vi "SubPanel_RunVI_Parameter.vi"(8 "error in (no error)":errorcluster, 9 "Values":variant[](array[variant]), 10 "Control Names":string[](array[string]), 11 "VIref in":refnum<vi>) -> (0 "error out":errorcluster, 3 "VIref out":refnum<vi>)   [LabVIEW 2014, in "SubPanelModule.lvlib"]
doc: "Imposta i controlli sul pannello del VI elencati da control names e Values.\nEsegue il VI solo se in Idle"
uses:
  <vilib>/Utility/error.llb/Error Cluster From Error Code.vi
  <vilib>/ErrorRing/Error Ring.xnode
  SubPanelModule.lvlib
panel:
  out "VI is RUN?":bool
  out "Exec.State":T1(ring)
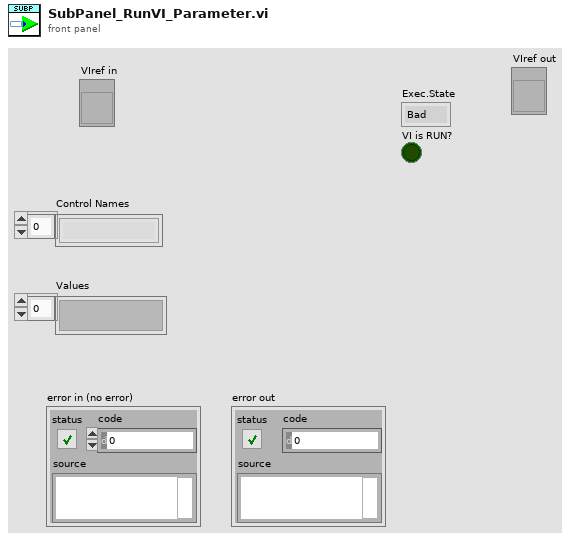
[diagram p1: front panel]
types:
  T1 = enum32{"Bad", "Idle", "Run top level", "Running"}
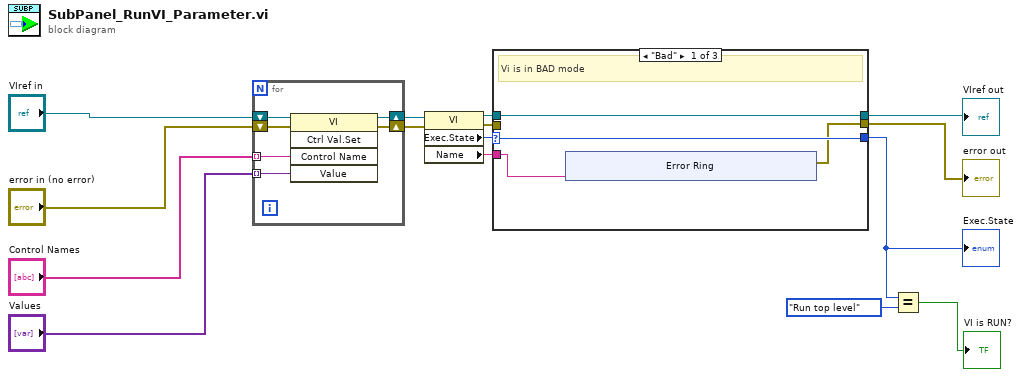
[diagram p0: block diagram]
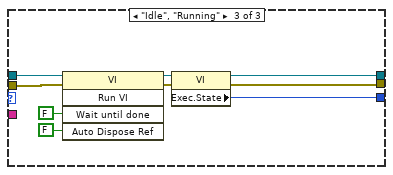
[diagram p3: hidden frame]
diagram:
  n1 = for {
    shift-right: [w19] -> w10
    shift-left: "VIref in" -> [w21]
    shift-right: [w20] -> w11
    shift-left: "error in (no error)" -> [w18]
    tunnel: "Control Names" -> [w17] mode=indexing
    tunnel: "Values" -> [w16] mode=indexing
    n2 = invoke class="VI" method="Ctrl Val.Set"(reference=w21, error in=w18, "Control Name"=w17, "Value"=w16) -> (reference out=w19:refnum<vi>, error out=w20:errorcluster)  [unwired: 1 in, 3 out]
  }
  n3 = property class="VI"(reference=w10, error in=w11) -> (reference out=w13:refnum<vi>, error out=w14:errorcluster, "Exec.State"=w12:T1, "Name"=w4:string)
  n4 = case shown="\"Bad\"" w12 {
    selector: w12 -> [w24 w33 _]
    tunnel: [w23 w35 w40] -> w8
    tunnel: w13 -> [w25 w34 w42]
    tunnel: w14 -> [_ w35 w41]
    tunnel: [w25 w34 w36] -> w5
    tunnel: [w24 w33 w37] -> w3
    tunnel: w4 -> [w22 _ _]
    frame "Bad" {
      # "Vi is in BAD mode"
      n5 = xnode "Error Ring"("parameter 0"=w22) -> ("error out"=w23:errorcluster)
    }
    frame "Run top level" {
      # "Vi is RUN - Do Nothing"
    }
    frame "Idle", "Running" {
      n6 = invoke class="VI" method="Run VI"(reference=w42, error in=w41, "Wait until done"=FALSE ("Wait Until Done"), "Auto Dispose Ref"=FALSE ("Auto Dispose Reference")) -> (reference out=w39:refnum<vi>, error out=w38:errorcluster)  [unwired: 1 in, 3 out]
      n7 = property class="VI"(reference=w39, error in=w38) -> (reference out=w36:refnum<vi>, error out=w40:errorcluster, "Exec.State"=w37:T1)
    }
  }
  "error out" <- w8
  "VIref out" <- w5
  "Exec.State" <- w3
  n8 = Equal?(x=w3, y=T1."Run top level") -> (x = y?=→"VI is RUN?":bool)
